vi "SetStagePosition.vi"(0 "Communication in":refnum<class "Microscope.lvclass">, 5 "Label":string, 7 "AbsPosition?":bool=TRUE, 9 "Value":dbl format="%#_13g", 11 "error in (no error)":errorcluster) -> (4 "Communication out":refnum<class "Microscope.lvclass">, 15 "error out":errorcluster)   [LabVIEW 2020, in "Microscope.lvlib" / "Microscope.lvclass"]
uses:
  Microscope.lvclass
  Microscope.lvclass/Microscope.ctl
  Component/Stage/Stage Messages/SetRelativePositionUm Msg/SetRelativePositionUm Msg.lvclass/SetRelativePositionUm Msg.ctl
  <vilib>/ActorFramework/Message Enqueuer/Message Enqueuer.lvclass/Message Enqueuer.ctl
  Component/Stage/Stage Messages/SetPositionUm Msg/SetPositionUm Msg.lvclass/SetPositionUm Msg.ctl
  <vilib>/ActorFramework/Message Enqueuer/Enqueue.vi
  Component/Stage/Stage Messages/SetRelativePositionUm Msg/SetRelativePositionUm Msg.lvclass
  C:/Program Files/National Instruments/LabVIEW 2020/vi.lib/ActorFramework/Message/Message.lvclass
  Component/Stage/Stage Messages/SetPositionUm Msg/SetPositionUm Msg.lvclass
  <vilib>/ActorFramework/Message Priority Queue/Priority Enqueue.vi
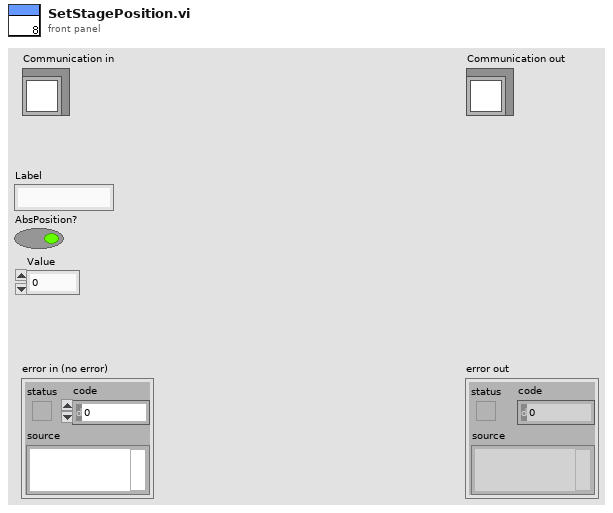
[diagram p1: front panel]
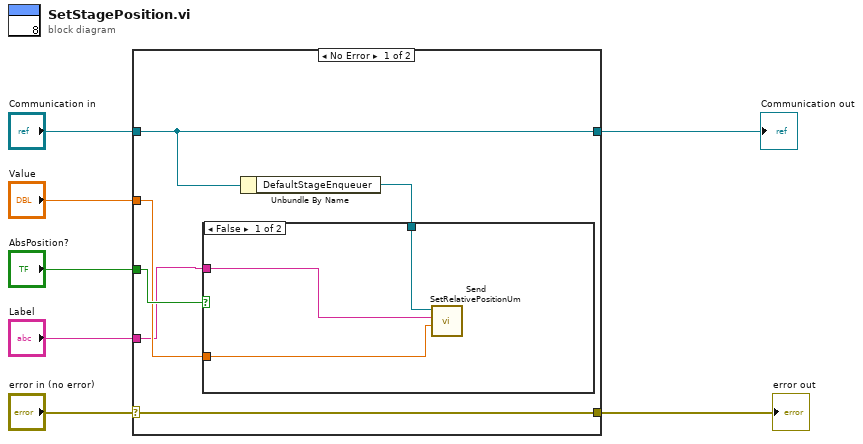
[diagram p0: block diagram]
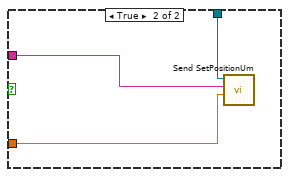
[diagram p2: hidden frame]
diagram:
  n1 = case shown="No Error" "error in (no error)" {
    selector: "error in (no error)" -> [w8 w21]
    tunnel: [w8 w21] -> w6
    tunnel: "Communication in" -> [w13 w20]
    tunnel: [w13 w20] -> w4
    tunnel: "Label" -> [w10 _]
    tunnel: "AbsPosition?" -> [w12 _]
    tunnel: "Value" -> [w11 _]
    frame No Error {
      n2 = Unbundle By Name(w13) -> ("DefaultStageEnqueuer"=w9:refnum<class "Message Enqueuer.lvclass">)
      n3 = case shown="False" w12 {
        tunnel: w11 -> [w14 w17]
        tunnel: w10 -> [w15 w18]
        tunnel: w9 -> [w16 w19]
        frame False {
          n4 = call "Send SetRelativePositionUm.vi"("RelativeMoveum"=w14, "Stage Label"=w15, "Message Enqueuer"=w16) -> ()  [unwired: 7 in, 2 out]
        }
        frame True {
          n5 = call "Send SetPositionUm.vi"("Positionum"=w17, "Stage Label"=w18, "Message Enqueuer"=w19) -> ()  [unwired: 7 in, 2 out]
        }
      }
    }
    frame Error {
    }
  }
  "error out" <- w6
  "Communication out" <- w4
